vi "Do Get Reference.vi"(8 "error in (no error)":errorcluster, 10 "Get Reference Argument":T2, 11 "Data Cluster in":T1) -> (0 "error out":errorcluster, 3 "Data Cluster out":T1)   [LabVIEW 2026, in "G-AI Core.lvlib"]
uses:
  G-AI Core.lvlib
  Module Data--cluster.ctl
  Get Reference Argument--cluster.ctl
  Get Reference (Reply Payload)--cluster.ctl
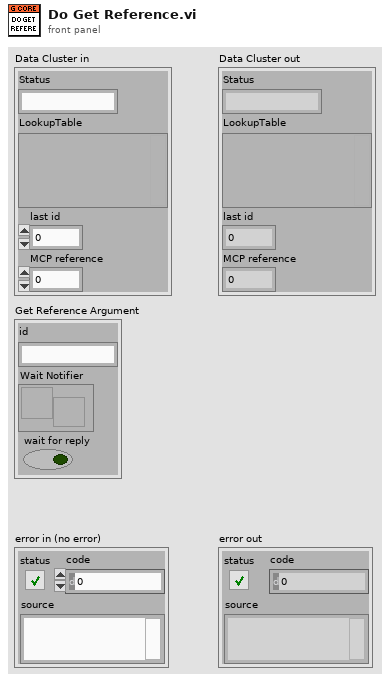
[diagram p1: front panel]
types:
  T1 = typedef "G-AI Core.lvlib/Module Data--cluster.ctl" = cluster{"Status":string, "LookupTable":variant, "last id":i32, "MCP reference":i32}
  T2 = typedef "G-AI Core.lvlib/Get Reference Argument--cluster.ctl" = cluster{"id":string, "Wait Notifier":refnum<notifier>, "wait for reply":bool}
  T3 = typedef "G-AI Core.lvlib/Get Reference (Reply Payload)--cluster.ctl" = cluster{"reference":variant, "error":errorcluster}
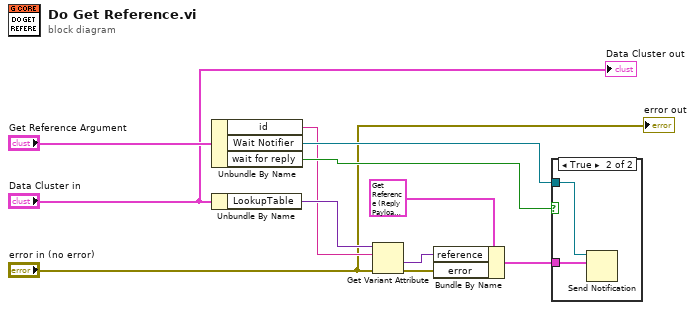
[diagram p0: block diagram]
diagram:
  n1 = Unbundle By Name("Get Reference Argument") -> ("id"=w4:string, "Wait Notifier"=w8:refnum<notifier>, "wait for reply"=w9:bool)
  n2 = Unbundle By Name("Data Cluster in") -> ("LookupTable"=w5:variant)
  n3 = Get Variant Attribute(Variant=w5, name=w4, error in="error in (no error)") -> (value=w1:variant, error out=w2:errorcluster)  [unwired: 1 in, 2 out]
  n4 = Bundle By Name(cluster=T3 {"reference"=variant, "error"={"status"=FALSE, "code"=0, "source"=""}} ("Get Reference (Reply Payload)"), "reference"=w1, "error"=w2) -> (w10:T3)
  n5 = case "DQMH_FIRE_NOTIFIER" shown="True" w9 {
    tunnel: w8 -> [_ w13]
    tunnel: w10 -> [_ w12]
    frame False {
    }
    frame True {
      n6 = Send Notification(notification=w12, notifier=w13) -> ()  [unwired: 1 in, 2 out]
    }
  }
  "Data Cluster out" <- "Data Cluster in"
  "error out" <- "error in (no error)"
